vi "isSharedResource.vi"(8 "error in (no error)":errorcluster, 11 "SMO in":refnum<class "SMO.lvclass">) -> (0 "error out":errorcluster, 2 "shared resource":bool, 3 "SMO out":refnum<class "SMO.lvclass">)   [LabVIEW 2021, in "smo.lvlib" / "SMO.lvclass"]
uses:
  SMO.lvclass
  Support/Attribute.SharedResource/Attribute.SharedResource.lvclass
  C:/Repositories/SMO/src/Support/Attribute/Attribute.lvclass
  SMO.lvclass/SMO.ctl
  C:/Repositories/SMO/src/Support/Attribute.SharedResource/Attribute.SharedResource.lvclass
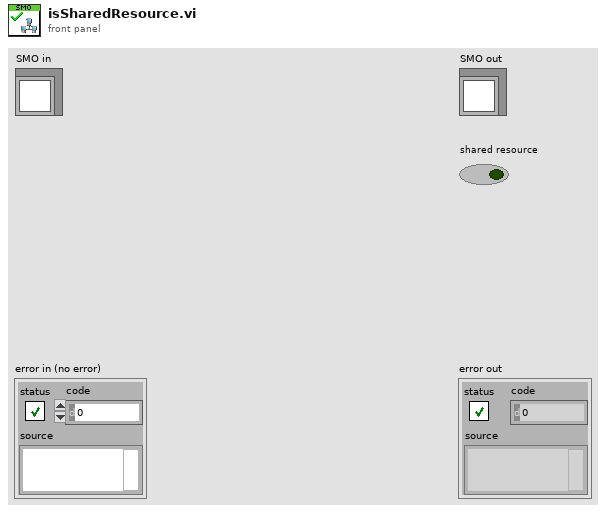
[diagram p1: front panel]
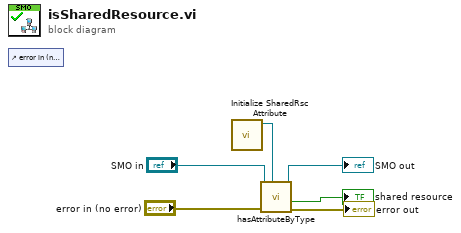
[diagram p0: block diagram]
diagram:
  n1 = control-ref of="error in (no error)"() -> ()  [unwired: 1 out]
  n2 = call "Initialize SharedRsc Attribute.vi"() -> ("Attribute.SharedResource"=w1:refnum<class "Attribute.SharedResource.lvclass">)  [unwired: 11 in]
  n3 = call "hasAttributeByType.vi"("Attribute Type"=w1, "error in (no error)"="error in (no error)", "SMO in"="SMO in") -> ("error out"=→"error out":errorcluster, "found"=→"shared resource":bool, "SMO in"=→"SMO out":refnum<class "SMO.lvclass">)  [unwired: 6 in]
